vi "Run.vi"(8 "error in (no error)":errorcluster, 9 "s on last turn":dbl, 10 "Maze (0: Empty, -1: Enemy. >0: Teammate":i32[][](array[numeric]), 11 "Explorer in":refnum<class "Explorer.lvclass">) -> (0 "error out":errorcluster, 1 "Direction":T1, 2 "Action":T2, 3 "Explorer out":refnum<class "Explorer.lvclass">, 4 "Replicated":refnum<class "Square.lvclass">)   [LabVIEW 2014, in "Explorer.lvclass"]
uses:
  Explorer.lvclass
  SquareBattle Arena/Action Enum.ctl
  SquareBattle Arena/Direction Enum.ctl
  Square.lvclass
  Explorer.lvclass/Explorer.ctl
  SquareBattle Arena/SquareBattle Arena.lvclass
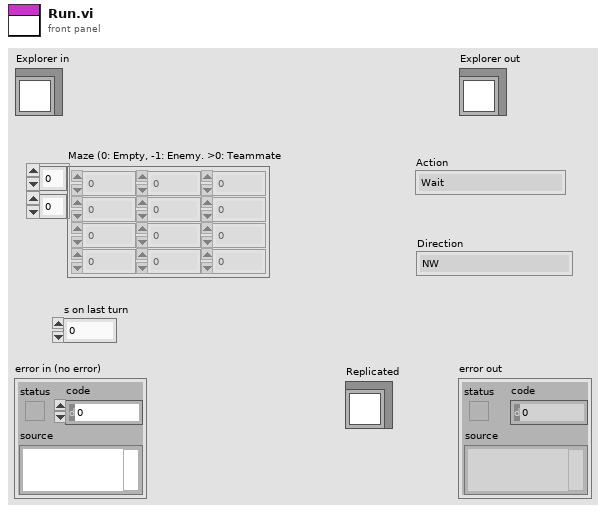
[diagram p1: front panel]
types:
  T1 = typedef "SquareBattle Arena.lvlib/SquareBattle Arena.lvclass/Direction Enum.ctl" = enum16{"NW", "N", "NE", "E", "SE", "S", "SW", "W"}
  T2 = typedef "SquareBattle Arena.lvlib/SquareBattle Arena.lvclass/Action Enum.ctl" = enum16{"Wait", "Move", "Attack", "Replicate"}
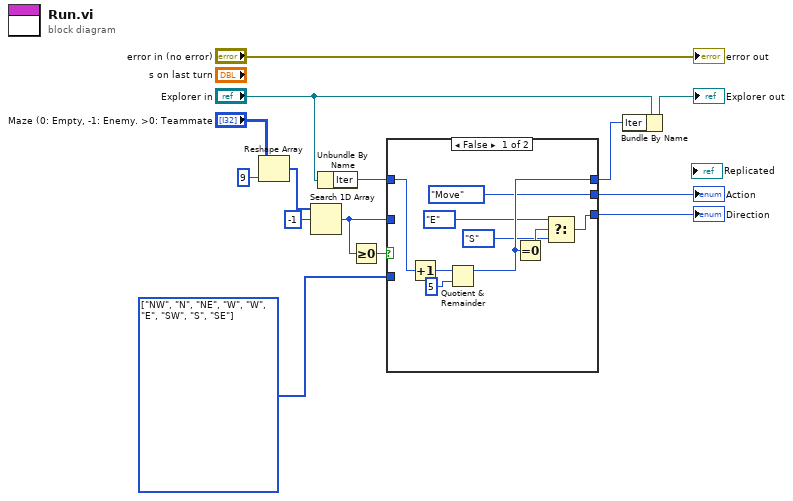
[diagram p0: block diagram]
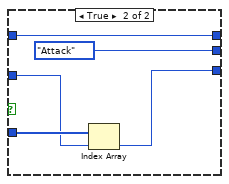
[diagram p2: hidden frame]
diagram:
  w4 = T1[] [enum."NW", enum."N", enum."NE", enum."W", enum."W", enum."E", enum."SW", enum."S", enum."SE"] items=["NW", "N", "NE", "E", "SE", "S", "SW", "W"]
  n1 = Reshape Array("Maze (0: Empty, -1: Enemy. >0: Teammate", 9 ("dimension size")) -> (w9:i32[])
  n2 = Search 1D Array(1D array=w9, element=-1) -> (index of element=w12:i32)  [unwired: 1 in]
  n3 = Unbundle By Name("Explorer in") -> ("Iter"=w6:i32)
  n4 = Greater Or Equal To 0?(x=w12) -> (x >= 0?=w11:bool)
  n5 = case shown="False" w11 {
    tunnel: [Action_Enum."Move" ("Action") Action_Enum."Attack" ("Action")] -> w2
    tunnel: w12 -> [_ w27]
    tunnel: w4 -> [_ w28]
    tunnel: [w20 w26] -> w3
    tunnel: w6 -> [w19 w24]
    tunnel: [w18 w24] -> w5
    frame False {
      n6 = Increment(x=w19) -> (x+1=w22:i32)
      n7 = Quotient & Remainder(x=w22, y=5 ("dimension size")) -> (x-y*floor(x/y)=w18:i32)  [unwired: 1 out]
      n8 = Equal To 0?(x=w18) -> (x = 0?=w21:bool)
      n9 = Select(t=Direction_Enum."E" ("Direction"), s=w21, f=Direction_Enum."S" ("Direction")) -> (s? t:f=w20:T1)
    }
    frame True {
      n10 = Index Array(array=w28, index=w27) -> (element=w26:T1)
    }
  }
  "Action" <- w2
  "Direction" <- w3
  n11 = Bundle By Name(cluster="Explorer in", "Iter"=w5) -> (→"Explorer out":refnum<class "Explorer.lvclass">)
  "error out" <- "error in (no error)"
